vi "选择启动参数.vi"() -> ()   [LabVIEW 2016, in "综合生物毒性.lvlib"]
uses:
  <vilib>/Utility/miscctls.llb/LVStringsAndValuesArrayTypeDef_U16.ctl
panel:
  in  "维护模式":bool=TRUE
  in  "取消":bool
  in  "确定":bool
  in  "站号":u16(ring)=1 items=["综合生物毒性"]
  in  "控制命令":T1(ring)
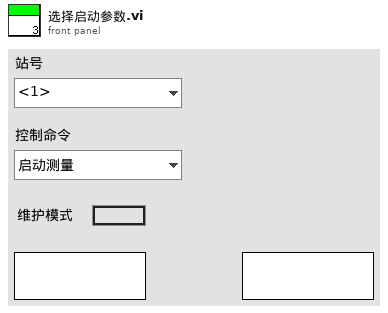
[diagram p1: front panel]
types:
  T1 = enum16{"启动测量", "标样核查", "零点核查", "跨度核查", "空白测试", "平行样测试", "加标回收", "空白校准", "标样校准", "初始化（清洗）", "停止测试", "仪器重启", "校时", "模式设置", "测量间隔设置"}
  T2 = typedef "LVStringsAndValuesArrayTypeDef_U16.ctl" = cluster{"String":string, "Value":u16}[]
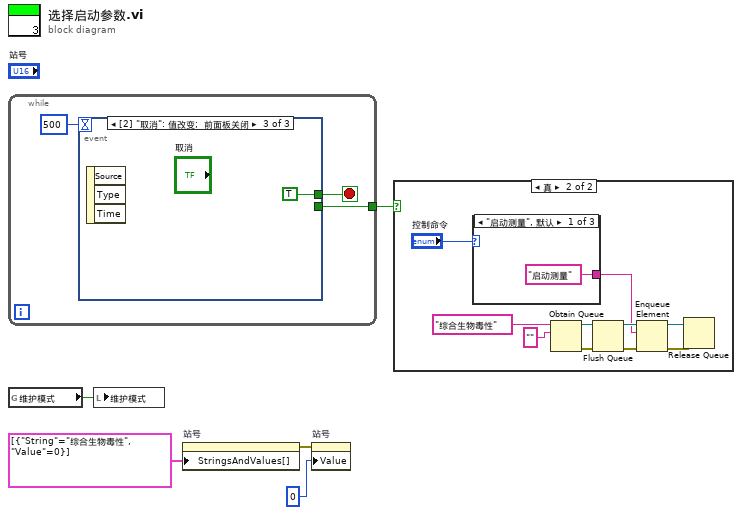
[diagram p0: block diagram]
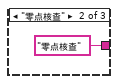
[diagram p3: hidden frame]
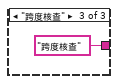
[diagram p4: hidden frame]
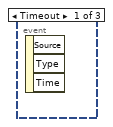
[diagram p5: hidden frame]
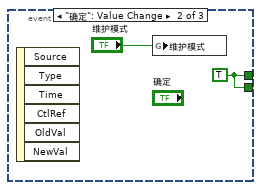
[diagram p6: hidden frame]
diagram:
  n1 = while {
    tunnel: [w7] -> w1
    stop <- w6 stop-if-true
    n2 = event shown="[2] \"取消\": 值改变;  前面板关闭" {
      selector: _ -> [_ _ _]
      dyn-events: _ -> [_ _ _]
      timeout: 500 -> [_ _ _]
      tunnel: [_ w9 _] -> w7
      tunnel: [_ w9 TRUE] -> w6
      event Timeout {
        n3 = event-data() -> ()  [unwired: 1 in, 3 out]
      }
      event "确定": Value Change {
        w9 = TRUE
        n4 = event-data() -> ()  [unwired: 1 in, 6 out]
        n5 = global write "VAR总磷总氮全局变量.vi" "维护模式"("维护模式") -> ()
      }
      event "取消": Value Change; Panel Close {
        n6 = event-data() -> ()  [unwired: 1 in, 3 out]
      }
    }
  }
  n7 = global read "VAR总磷总氮全局变量.vi" "维护模式"() -> (w2:bool)
  n8 = local write "维护模式"(w2) -> ()
  n9 = property on="站号" class="Ring (严格)"("StringsAndValues[]"=T2 [{"String"="综合生物毒性", "Value"=0}] ("字符串与值[]")) -> (error out=w4:errorcluster)  [unwired: 2 in, 1 out]
  n10 = property on="站号" class="Ring (严格)"(error in=w4, "Value"=0) -> ()  [unwired: 1 in, 2 out]
  n11 = case shown="真" w1 {
    frame False {
    }
    frame True {
      n12 = case shown="\"启动测量\", 默认" "控制命令" {
        tunnel: ["启动测量" ("元素") "零点核查" ("元素") "跨度核查" ("元素")] -> w14
        frame "启动测量", Default {
        }
        frame "零点核查" {
        }
        frame "跨度核查" {
        }
      }
      n13 = Obtain Queue(name (unnamed)="综合生物毒性" ("名称（未命名）"), element data type="" ("状态")) -> (queue out=w18:refnum<queue>, error out=w17:errorcluster)  [unwired: 3 in, 1 out]
      n14 = Flush Queue(queue=w18, error in (no error)=w17) -> (queue out=w16:refnum<queue>, error out=w15:errorcluster)  [unwired: 1 out]
      n15 = Enqueue Element(queue=w16, element=w14, error in (no error)=w15) -> (queue out=w13:refnum<queue>, error out=w12:errorcluster)  [unwired: 1 in, 1 out]
      n16 = Release Queue(queue=w13, error in (no error)=w12) -> ()  [unwired: 1 in, 3 out]
    }
  }
